vi "ELMOS Start Prog.vi"(9 "AppFileName":string, 10 "LINChannel":u8, 11 "DeviceHandle":i32) -> (3 "function return":i32)   [LabVIEW 2010, in "elmos_programer.lvlib"]
doc: "int WINAPI ELMOS_StartProg(int DeviceHandle, unsigned char LINChannel,const char* AppFileName);"
uses:
  elmos_programer.lvlib
  USB2XXX/trunk/USB2XXX/USB2XXX/vs2019/Release/USB2XXX.dll
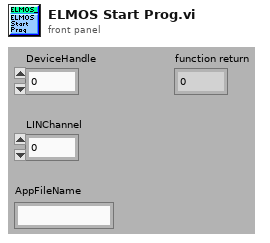
[diagram p1: front panel]
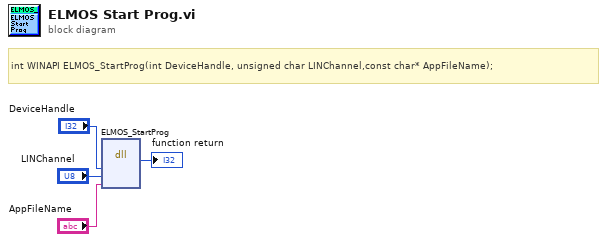
[diagram p0: block diagram]
diagram:
  # "int WINAPI ELMOS_StartProg(int DeviceHandle, unsigned char LINChannel,const char* AppFileName);"
  n1 = dll-call lib="E:/Projects/USB2XXX/trunk/USB2XXX/USB2XXX/vs2019/Release/USB2XXX.*" fn="ELMOS_StartProg"("DeviceHandle"="DeviceHandle", "LINChannel"="LINChannel", "AppFileName"="AppFileName") -> (→"function return":i32)  [unwired: 6 in, 2 out]
